vi "Draw+2.vi"(2 "Color":u32(colorbox)=16711680, 3 "H":i32, 4 "W":i32, 5 "input cluster":cluster{"P_X":i32, "P_Y":i32}, 6 "Image In":T1) -> (0 "Image Out":T1)   [LabVIEW 2014]
uses:
  <vilib>/vision/Image Controls.llb/IMAQ Image.ctl
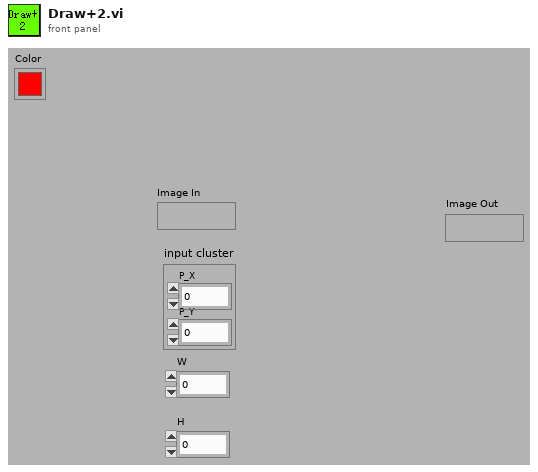
[diagram p1: front panel]
types:
  T1 = typedef "IMAQ Image.ctl" = refnum<image>
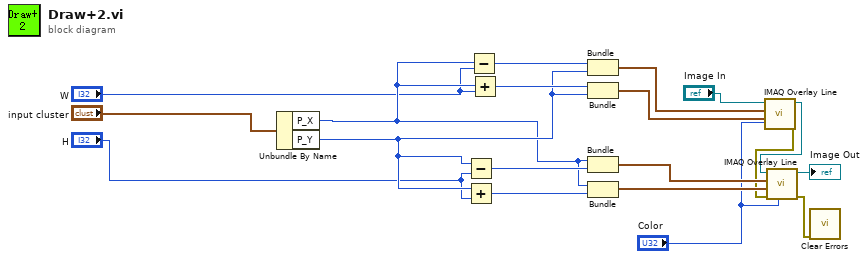
[diagram p0: block diagram]
diagram:
  n1 = Unbundle By Name("input cluster") -> ("P_X"=w10:i32, "P_Y"=w14:i32)
  n2 = Subtract(x=w14, y="H") -> (x-y=w12:i32)
  n3 = Add(x=w14, y="H") -> (x+y=w11:i32)
  n4 = Subtract(x=w10, y="W") -> (x-y=w18:i32)
  n5 = Add(x=w10, y="W") -> (x+y=w15:i32)
  n6 = Bundle(w18, "P_Y"=w14) -> (w16:cluster{i32, "P_Y":i32})  [unwired: 1 in]
  n7 = Bundle(w15, "P_Y"=w14) -> (w13:cluster{i32, "P_Y":i32})  [unwired: 1 in]
  n8 = Bundle("P_X"=w10, w12) -> (w8:cluster{"P_X":i32, i32})  [unwired: 1 in]
  n9 = Bundle("P_X"=w10, w11) -> (w7:cluster{"P_X":i32, i32})  [unwired: 1 in]
  n10 = call "IMAQ Overlay Line"("Color"="Color", "End Point"=w13, "Start Point"=w16, "Image"="Image In") -> ("error out"=w3:errorcluster, "Image Out"=w9:T1)  [unwired: 6 in]
  n11 = call "IMAQ Overlay Line"("Color"="Color", "error in (no error)"=w3, "End Point"=w7, "Start Point"=w8, "Image"=w9) -> ("error out"=w4:errorcluster, "Image Out"=→"Image Out":T1)  [unwired: 5 in]
  n12 = call <vilib>:"Clear Errors.vi"("error in (no error)"=w4) -> ()  [unwired: 5 in, 2 out]
